vi "RMS.vi"(11 "current waveform":waveform(dbl)) -> (3 "RMS":dbl)   [LabVIEW 2017]
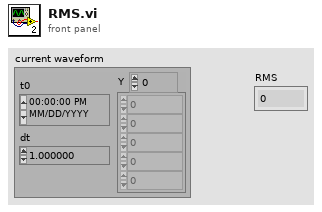
[diagram p1: front panel]
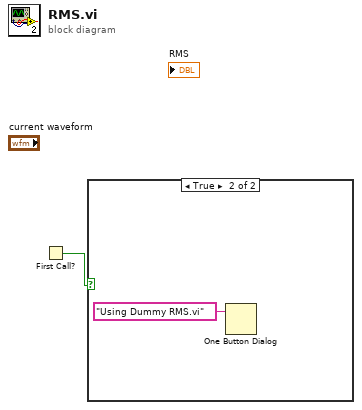
[diagram p0: block diagram]
diagram:
  n1 = First Call?() -> (First Call?: T/F=w1:bool)
  n2 = case shown="True" w1 {
    frame False {
    }
    frame True {
      n3 = One Button Dialog(message="Using Dummy RMS.vi") -> ()  [unwired: 1 in, 1 out]
    }
  }
